vi "niFpgaFFTStreamingOutputControlLogic.vi"(0 "reset":bool, 1 "process state in":enum8{"process", "idle"}(ring), 5 "ready for output":bool, 7 "execution constants":cluster{"bitmask":u16, "K-16":i8}) -> (3 "process state out":enum8{"process", "idle"}(ring), 4 "ready for input":bool, 6 "read address 0":u16, 8 "use buffer 0":bool, 10 "read address 1":u16, 13 "output valid":bool, 14 "data index":u16)   [LabVIEW 2017]
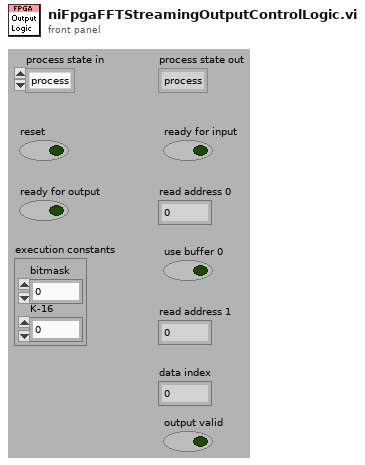
[diagram p1: front panel]
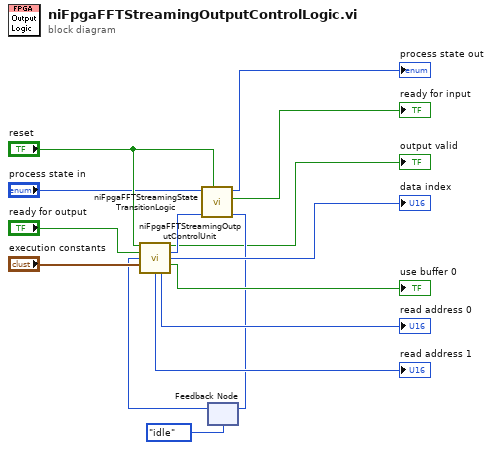
[diagram p0: block diagram]
diagram:
  n1 = feedback #1(enum8{"idle", "output"}."idle") -> (w3:enum8{"idle", "output"})
  n2 = call <vilib>:"niFpgaFFTStreamingOutputControlUnit.vi"("reset"="reset", "ready for output"="ready for output", "current status"=w3, "execution constants"="execution constants") -> ("output valid (inside)"=→"output valid":bool, "next status"=w8:enum8{"idle", "output"}, "data index"=→"data index":u16, "use buffer 0"=→"use buffer 0":bool, "read address 1"=→"read address 1":u16, "read address 0"=→"read address 0":u16)  [unwired: 1 in, 5 out]
  n3 = call <vilib>:"niFpgaFFTStreamingStateTransitionLogic.vi"("reset"="reset", "output state in"=w8, "process state in"="process state in") -> ("output state out"=w7:enum8{"idle", "output"}, "ready for input"=→"ready for input":bool, "process state out"=→"process state out":enum8{"process", "idle"})  [unwired: 4 in, 2 out]
  n4 = feedback-in #1(w7) -> ()
